vi "Save Vel, Acc - Traj adj.vi"(2 "Vel,Acc graphs":string, 3 "Vel,Acc traj Adj data":string, 5 "Step":dbl, 7 "Animal Number":dbl, 8 "Velocity-Acceleration graphs":dbl[][](array[numeric]), 9 "Vel, Accel RMS":dbl[][](array[numeric]), 10 "#Crossings":i32[][](array[numeric]), 11 "Vel, Acc data":dbl[][](array[numeric])) -> ()   [LabVIEW 2020]
panel:
  out "concatenated string 3":string
  out "concatenated string 2":string
  out "Velocity-Acc graphs":dbl[][](array[numeric])
  out "Vel, Acc data":dbl[][](array[numeric])
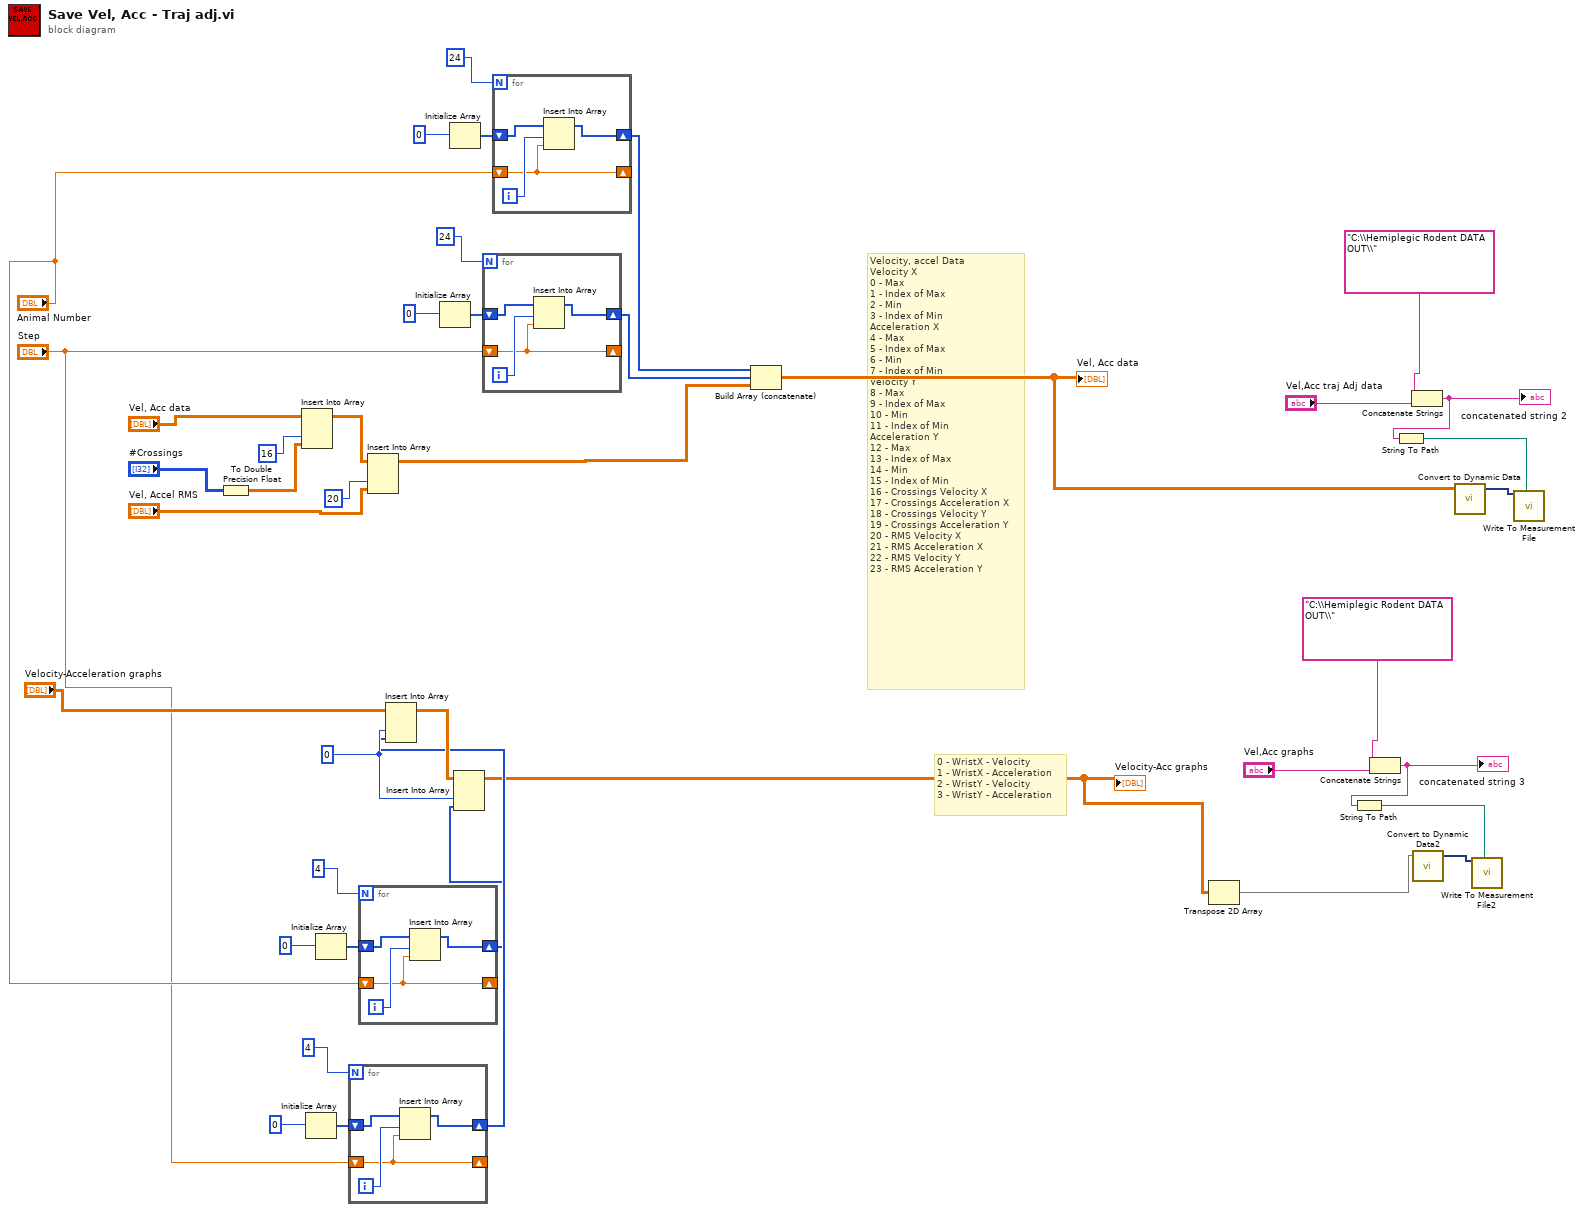
[diagram p0: block diagram]
diagram:
  w27 = 0
  # "0 - WristX - Velocity\n1 - WristX - Acceleration\n2 - WristY - Velocity\n3 - WristY - Acceleration"
  # "Velocity, accel Data\nVelocity X\n0 - Max\n1 - Index of Max\n2 - Min\n3 - Index of Min\nAcceleration X\n4 - Max\n5 - Index of Max\n6 - Min\n7 - Index of Min\nVelocity Y\n8 - Max\n9 - Index of Max\n10 - Min\n11 - Index of Min\nAcceleration Y\n12 - Max\n13 - Index of Max\n14 - Min\n15 - Index of Min\n16 - Crossings Velocity X\n17 - Crossings Acceleration X\n18 - Crossings Velocity Y\n19 - Crossings Acceleration Y\n20 - RMS Velocity X\n21 - RMS Acceleration X\n22 - RMS Velocity Y\n23 - RMS Acceleration Y"
  n1 = To Double Precision Float(number="#Crossings") -> (double precision float=w14:dbl[][])
  n2 = Insert Into Array(array="Vel, Acc data", index (col)=16, new element=w14) -> (w40:dbl[][])  [unwired: 1 in]
  n3 = Initialize Array(0) -> (w20:i32[])  [unwired: 1 in]
  n4 = Initialize Array(0) -> (w23:i32[])  [unwired: 1 in]
  n5 = for {
    N: 4 -> [_]
    shift-right: [w44] -> w17
    shift-left: w20 -> [w45]
    shift-right: [w43] -> _
    shift-left: "Step" -> [w43]
    i -> [w46]
    n6 = Insert Into Array(array=w45, index=w46, new element=w43) -> (w44:i32[])
  }
  n7 = for {
    N: 4 -> [_]
    shift-right: [w48] -> w16
    shift-left: w23 -> [w49]
    shift-right: [w47] -> _
    shift-left: "Animal Number" -> [w47]
    i -> [w50]
    n8 = Insert Into Array(array=w49, index=w50, new element=w47) -> (w48:i32[])
  }
  n9 = Insert Into Array(array=w40, index (col)=20, new element="Vel, Accel RMS") -> (w30:dbl[][])  [unwired: 1 in]
  n10 = Insert Into Array(array="Velocity-Acceleration graphs", index (col)=w27, new element=w17) -> (w26:dbl[][])  [unwired: 1 in]
  n11 = Initialize Array(0) -> (w33:i32[])  [unwired: 1 in]
  n12 = Initialize Array(0) -> (w36:i32[])  [unwired: 1 in]
  n13 = Insert Into Array(array=w26, index (col)=w27, new element=w16) -> (w2:dbl[][])  [unwired: 1 in]
  "Velocity-Acc graphs" <- w2
  n14 = for {
    N: 24 -> [_]
    shift-right: [w52] -> w31
    shift-left: w33 -> [w53]
    shift-right: [w51] -> _
    shift-left: "Step" -> [w51]
    i -> [w54]
    n15 = Insert Into Array(array=w53, index=w54, new element=w51) -> (w52:i32[])
  }
  n16 = for {
    N: 24 -> [_]
    shift-right: [w56] -> w32
    shift-left: w36 -> [w57]
    shift-right: [w55] -> _
    shift-left: "Animal Number" -> [w55]
    i -> [w58]
    n17 = Insert Into Array(array=w57, index=w58, new element=w55) -> (w56:i32[])
  }
  n18 = Build Array (concatenate)(w32, w31, w30) -> (w8:dbl[][])
  "Vel, Acc data" <- w8
  n19 = Transpose 2D Array(2D array=w2) -> (transposed array=w1:dbl[][])
  n20 = Concatenate Strings("C:\\Hemiplegic Rodent DATA OUT\\" ("name"), "Vel,Acc graphs") -> (w6:string)
  "concatenated string 3" <- w6
  n21 = String To Path(string=w6) -> (path=w4:path)
  n22 = Concatenate Strings("C:\\Hemiplegic Rodent DATA OUT\\" ("name"), "Vel,Acc traj Adj data") -> (w12:string)
  "concatenated string 2" <- w12
  n23 = String To Path(string=w12) -> (path=w10:path)
  n24 = call "Convert to Dynamic Data2"("2D Array"=w1) -> ("Dynamic Data Type"=w3:dynamicdata)  [unwired: 3 in]
  n25 = call "Convert to Dynamic Data"("2D Array"=w8) -> ("Dynamic Data Type"=w9:dynamicdata)  [unwired: 3 in]
  n26 = call "Write To Measurement File2"("Signals"=w3, "Filename"=w4) -> ()  [unwired: 15 in, 3 out]
  n27 = call "Write To Measurement File"("Signals"=w9, "Filename"=w10) -> ()  [unwired: 15 in, 3 out]
